vi "Read.vi"(8 "error in (no error)":errorcluster, 11 "State in":refnum<class "State.lvclass">) -> (0 "error out":errorcluster, 2 "state data":T1, 3 "State out":refnum<class "State.lvclass">)   [LabVIEW 2017, in "DSF Core.lvlib" / "State.lvclass"]
uses:
  State.lvclass
  State Data.ctl
  State.lvclass/State.ctl
  <vilib>/NI/Memory Manager/Classes/Pointer/Pointer.lvclass/Pointer.ctl
  <vilib>/NI/Memory Manager/Classes/Pointer/Pointer.lvclass
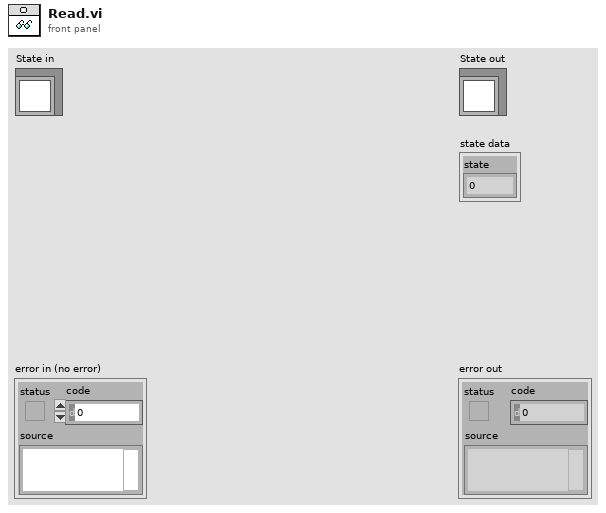
[diagram p1: front panel]
types:
  T1 = typedef "DSF Core.lvlib/State.lvclass/State Data.ctl" = cluster{"state":u8}
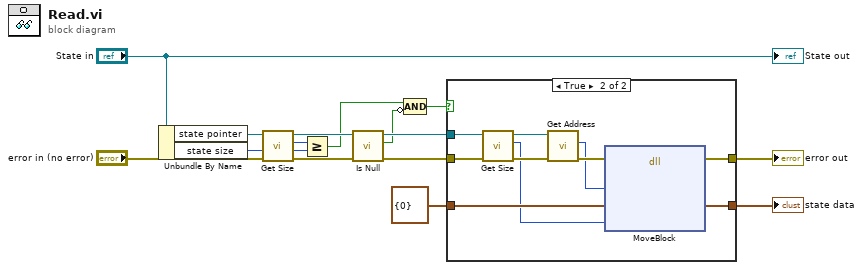
[diagram p0: block diagram]
diagram:
  n1 = Unbundle By Name("State in") -> ("state pointer"=w11:refnum<class "Pointer.lvclass">, "state size"=w10:u64)
  n2 = call <vilib>:"Get Size.vi"("Pointer in"=w11) -> ("size"=w8:u64, "Pointer out"=w9:refnum<class "Pointer.lvclass">)  [unwired: 9 in]
  n3 = Greater Or Equal?(x=w8, y=w10) -> (x >= y?=w7:bool)
  n4 = call <vilib>:"Is Null.vi"("error in (no error)"="error in (no error)", "Pointer in"=w9) -> ("error out"=w4:errorcluster, "null?"=w3:bool, "Pointer out"=w5:refnum<class "Pointer.lvclass">)  [unwired: 7 in]
  n5 = Compound Arithmetic op=AND(w7, invert w3) -> (w6:bool)
  n6 = case shown="True" w6 {
    tunnel: w5 -> [_ w22]
    tunnel: w4 -> [w16 w24]
    tunnel: [w16 w20] -> w14
    tunnel: [w15 w19] -> w2
    tunnel: T1 {"state"=0} ("state data") -> [w15 w18]
    frame False {
    }
    frame True {
      n7 = call <vilib>:"Get Size.vi"("Pointer in"=w22) -> ("size"=w17:u64, "Pointer out"=w21:refnum<class "Pointer.lvclass">)  [unwired: 9 in]
      n8 = call <vilib>:"Get Address.vi"("Pointer in"=w21) -> ("address"=w23:u64)  [unwired: 9 in, 1 out]
      n9 = dll-call lib="LabVIEW" fn="MoveBlock"(error in=w24, "src"=w23, "dst"=w18, "size"=w17) -> (error out=w20:errorcluster, "dst"=w19:T1)  [unwired: 5 in, 1 out]
    }
  }
  "error out" <- w14
  "state data" <- w2
  "State out" <- "State in"
